vi "Get Encoder Parameters.vi"() -> (0 "Encoder Offset":i32, 2 "Encoder Scale":u32, 3 "Encoder Size":u16)   [LabVIEW 2015, in "Tool Cfg.lvlib"]
uses:
  Tool Cfg.lvlib
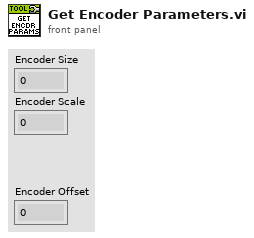
[diagram p1: front panel]
types:
  T1 = typedef "Tool Cfg.lvlib/_Tool Block Cluster--typedef.ctl" = cluster{"Encoder Size":u16, "Encoder Scale":u32, "Encoder Offset":i32, "MaxEncoder":i32, "MinEncoder":i32, "Start Delay":sgl}
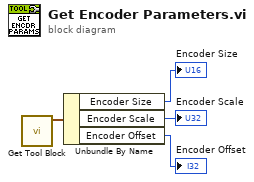
[diagram p0: block diagram]
diagram:
  n1 = call "Get Tool Block.vi"() -> ("Tool Block"=w4:T1)  [unwired: 11 in]
  n2 = Unbundle By Name(w4) -> ("Encoder Size"=→"Encoder Size":u16, "Encoder Scale"=→"Encoder Scale":u32, "Encoder Offset"=→"Encoder Offset":i32)
